vi "陀螺状态自检.vi"(10 "G123":string, 11 "陀螺自检状态字":u8) -> (3 "连接的字符串":string)   [LabVIEW 2012]
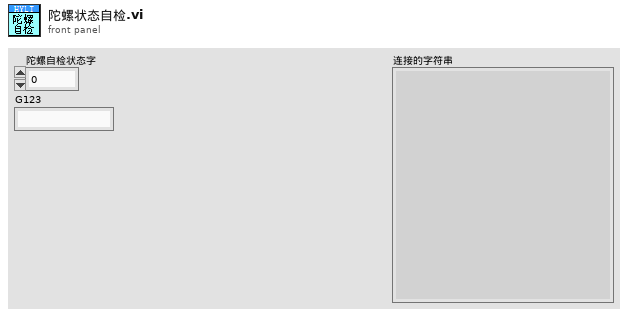
[diagram p1: front panel]
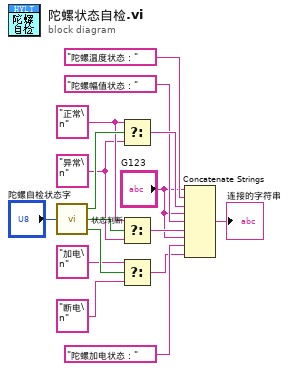
[diagram p0: block diagram]
diagram:
  w10 = "异常\n" ("f")
  w11 = "正常\n" ("主份自检状态及船舱标志")
  n1 = call "状态判断.vi"("数值"="陀螺自检状态字") -> ("D0"=w14:bool, "D01"=w13:bool, "D02"=w12:bool)
  n2 = Select(t=w11, s=w14, f=w10) -> (s? t:f=w7:string)
  n3 = Select(t=w11, s=w13, f=w10) -> (s? t:f=w5:string)
  n4 = Select(t="加电\n" ("f"), s=w12, f="断电\n") -> (s? t:f=w3:string)
  n5 = Concatenate Strings("G123", "陀螺温度状态：" ("字符串"), w7, "G123", "陀螺幅值状态：" ("字符串"), w5, "G123", "陀螺加电状态：" ("字符串"), w3) -> (→"连接的字符串":string)
